vi "Set Out.vi"(8 "error in (no error)":errorcluster, 10 "Output value":refnum<class "Output Value.lvclass">, 11 "CS580 Driver in":refnum<class "CS580 Driver.lvclass">) -> (0 "error out":errorcluster, 3 "CS580 Driver out":refnum<class "CS580 Driver.lvclass">)   [LabVIEW 2025, in "CS580 Driver.lvclass"]
uses:
  CS580 Driver.lvclass
  C:/GitHub/NHMFL_Core/Libraries/Instruments/VISA Instrument/VISA Instrument.lvclass
  Utilities/Output Value/Output Value.lvclass
  C:/GitHub/NHMFL_Core/Libraries/Instruments/Results/Acquired Result/Acquired Result.lvclass
  VISA Instrument/VISA Instrument.lvclass/VISA Instrument.ctl
  CS580 Driver.lvclass/CS580 Driver.ctl
  VISA Instrument/Read VISA resource.vi
  VISA Instrument/Write VISA resource.vi
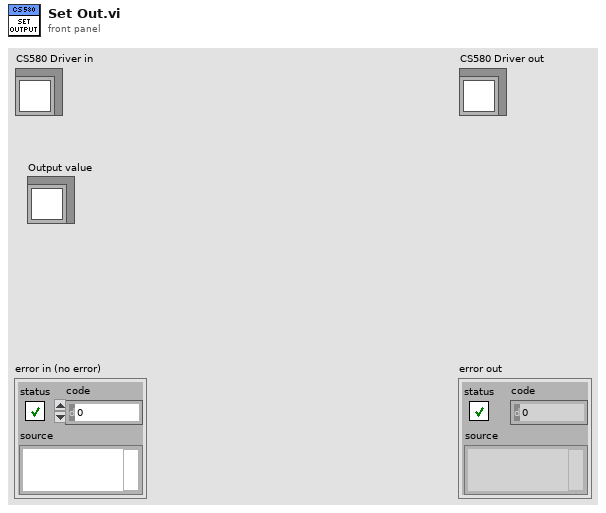
[diagram p1: front panel]
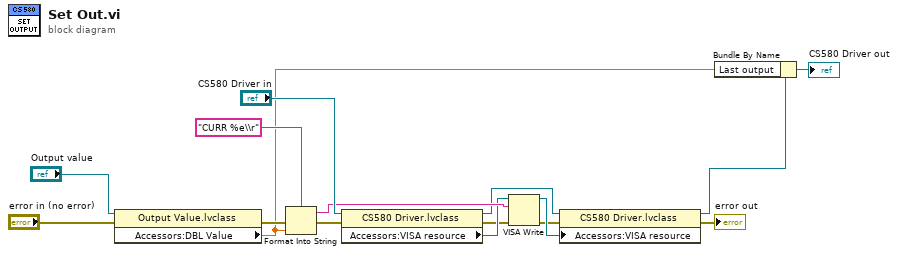
[diagram p0: block diagram]
diagram:
  n1 = property class="Output Value.lvclass"(reference="Output value", error in="error in (no error)") -> (error out=w13:errorcluster, "Accessors:DBL Value"=w1:dbl)  [unwired: 1 out]
  n2 = Format Into String(format string="CURR %e\\r", error in=w13, w1) -> (resulting string=w10:string, error out=w12:errorcluster)  [unwired: 1 in]
  n3 = property class="CS580 Driver.lvclass"(reference="CS580 Driver in", error in=w12) -> (reference out=w9:refnum<class "CS580 Driver.lvclass">, error out=w6:errorcluster, "Accessors:VISA resource"=w7:refnum<visa-resource-name>)
  n4 = VISA Write(VISA resource name=w7, write buffer=w10, error in (no error)=w6) -> (VISA resource name out=w8:refnum<visa-resource-name>, error out=w5:errorcluster)  [unwired: 1 out]
  n5 = property class="CS580 Driver.lvclass"(reference=w9, error in=w5, "Accessors:VISA resource"=w8) -> (reference out=w3:refnum<class "CS580 Driver.lvclass">, error out=→"error out":errorcluster)
  n6 = Bundle By Name(cluster=w3, "Last output"=w1) -> (→"CS580 Driver out":refnum<class "CS580 Driver.lvclass">)
